vi "read_bin.vi"(4 "error in":errorcluster, 7 "datalog path":path) -> (0 "error out":errorcluster, 1 "Waveform Graph":waveform(i16)[](graph), 2 "group name":string, 3 "new file path":path)   [LabVIEW 2010]
panel:
  out "t0":timestamp format="%<%.6X\n%x>T"
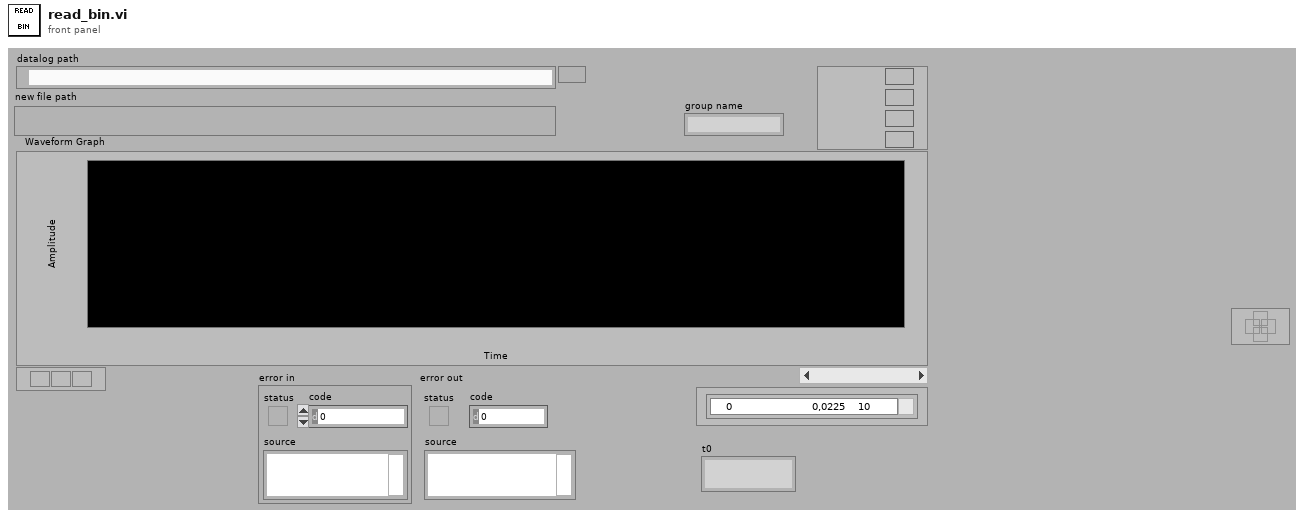
[diagram p1: front panel]
types:
  T1 = enum16{"open", "open or create", "create or replace", "create", "open (read-only)"}
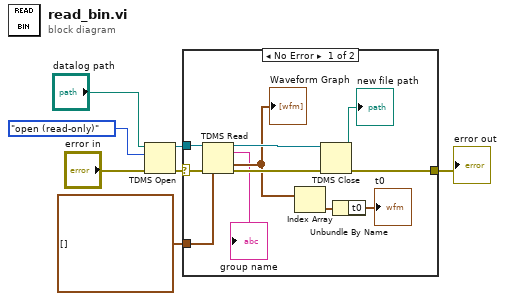
[diagram p0: block diagram]
diagram:
  n1 = TDMS Open(8:"error in", 10:T1."open (read-only)" ("operation (0:open)"), 11:"datalog path") -> (0:w3:errorcluster, 3:w7:refnum<k34>)  [unwired: 3 in]
  n2 = case shown="No Error" w3 {
    selector: w3 -> [w10 w19]
    tunnel: w7 -> [w16 _]
    tunnel: [w11 w19] -> w2
    tunnel: waveform(i16)[] [] ("Array") -> [w9 _]
    frame No Error {
      n3 = TDMS Read(0:w16, 11:w10, 12:w9) -> (4:w14:refnum<k34>, 6:→"group name":string, 10:w13:waveform(i16)[], 15:w15:errorcluster)  [unwired: 4 in, 2 out]
      "Waveform Graph" <- w13
      n4 = Index Array(array=w13) -> (element=w18:waveform(i16))  [unwired: 1 in]
      n5 = TDMS Close(8:w15, 11:w14) -> (0:w11:errorcluster, 3:→"new file path":path)
      n6 = Unbundle By Name(w18) -> ("t0"=→"t0":timestamp)
    }
    frame Error {
    }
  }
  "error out" <- w2
